vi "test.vi"() -> ()   [LabVIEW 2015]
panel:
  out "error out":errorcluster
  in  "Cluster":cluster{}
  in  "Boolean 2":bool
  in  "String 2":string
  in  "Numeric 2":i32
  in  "String":string
  in  "Numeric":i32
  in  "Boolean":bool=TRUE
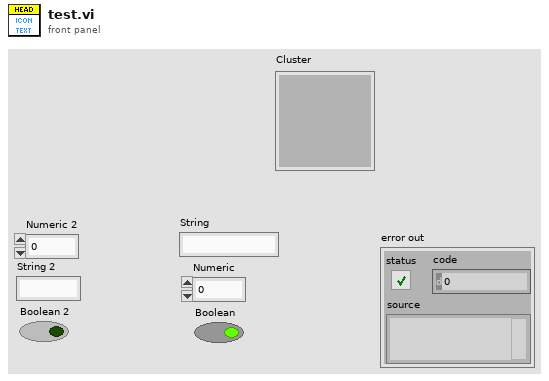
[diagram p1: front panel]
types:
  T1 = cluster{"String":string, "Numeric":i32, "Boolean":bool}
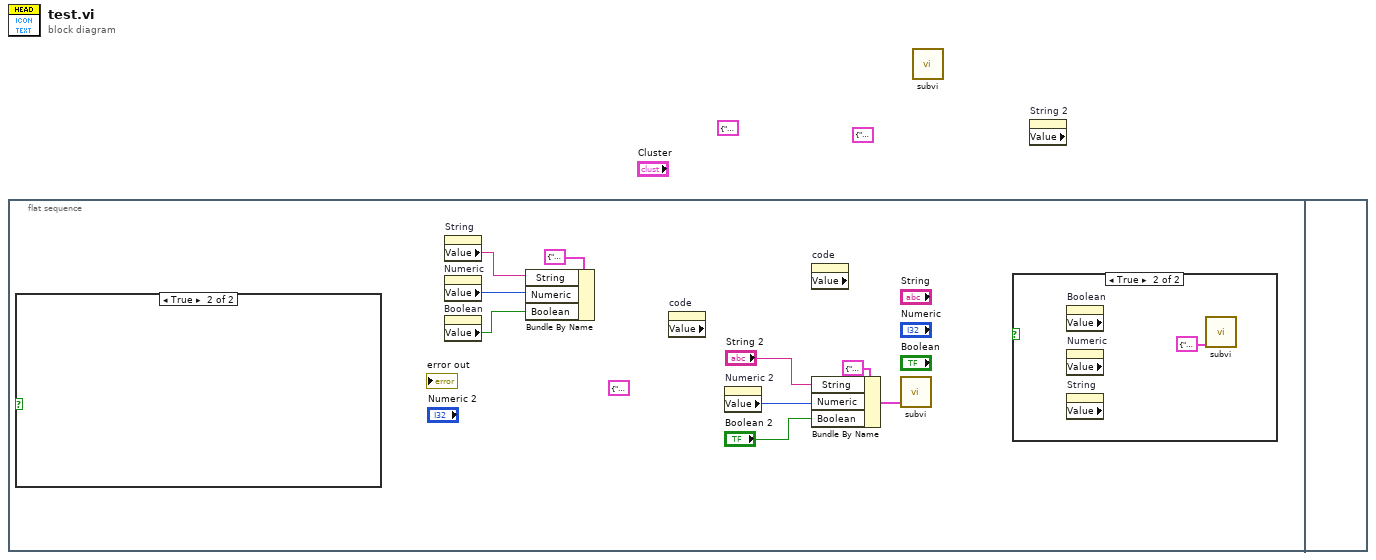
[diagram p0: block diagram]
diagram:
  (unwired) T1 {"String"="", "Numeric"=0, "Boolean"=FALSE} ("cluster in")
  (unwired) T1 {"String"="", "Numeric"=0, "Boolean"=FALSE} ("cluster in")
  n1 = flat-sequence {
    frame #0 {
      (unwired) T1 {"String"="", "Numeric"=0, "Boolean"=FALSE} ("cluster in")
      n2 = case shown="True" {
        selector: _ -> [_ _]
        frame False {
        }
        frame True {
        }
      }
      n3 = property on="String" class="Str"() -> ("Value"=w8:string)  [unwired: 2 in, 2 out]
      n4 = property on="Numeric" class="DigNum (strict)"() -> ("Value"=w9:i32)  [unwired: 2 in, 2 out]
      n5 = property on="Boolean" class="Bool (strict)"() -> ("Value"=w7:bool)  [unwired: 2 in, 2 out]
      n6 = Bundle By Name(cluster=T1 {"String"="", "Numeric"=0, "Boolean"=FALSE} ("cluster in"), "String"=w8, "Numeric"=w9, "Boolean"=w7) -> ()  [unwired: 1 out]
      n7 = property on="code" class="DigNum (strict)" props=["Value"]() -> ()  [unwired: 2 in, 3 out]
      n8 = property on="Numeric 2" class="DigNum (strict)"() -> ("Value"=w2:i32)  [unwired: 2 in, 2 out]
      n9 = property on="code" class="DigNum (strict)" props=["Value"]() -> ()  [unwired: 2 in, 3 out]
      n10 = Bundle By Name(cluster=T1 {"String"="", "Numeric"=0, "Boolean"=FALSE} ("cluster in"), "String"="String 2", "Numeric"=w2, "Boolean"="Boolean 2") -> (w5:T1)
      n11 = call "subvi.vi"("cluster in"=w5) -> ()  [unwired: 9 in, 2 out]
      n12 = case shown="True" {
        selector: _ -> [_ _]
        frame False {
        }
        frame True {
          n13 = property on="Boolean" class="Bool (strict)" props=["Value"]() -> ()  [unwired: 2 in, 3 out]
          n14 = property on="Numeric" class="DigNum (strict)" props=["Value"]() -> ()  [unwired: 2 in, 3 out]
          n15 = property on="String" class="Str" props=["Value"]() -> ()  [unwired: 2 in, 3 out]
          n16 = call "subvi.vi"("cluster in"=T1 {"String"="", "Numeric"=0, "Boolean"=FALSE}) -> ()  [unwired: 9 in, 2 out]
        }
      }
    }
    frame #1 {
    }
  }
  n17 = call "subvi.vi"() -> ()  [unwired: 10 in, 2 out]
  n18 = property on="String 2" class="Str" props=["Value"]() -> ()  [unwired: 2 in, 3 out]
